vi "rqcBob Initiate.vi"(0 "rqcBob in":refnum<class "rqcBob.lvclass">, 11 "error in (no error)":errorcluster) -> (4 "rqcBob out":refnum<class "rqcBob.lvclass">, 15 "error out":errorcluster)   [LabVIEW 2018, in "rqcBob.lvclass"]
uses:
  rqcBob.lvclass
  rqcBob.lvclass/rqcBob.ctl
  Custom Controls/rqcBob Main FPGA interface.ctl
  Custom Controls/rqcBob State.ctl
  <vilib>/Utility/error.llb/Error Cluster From Error Code.vi
  <vilib>/rvi/errors/niLvFpgaAdjustHostInterfaceError.vi
  <vilib>/rvi/interface/nirviReadWriteControl/nirviReadWriteControl.xnode
  NiFpgaLv.dll
  <vilib>/rvi/interface/Simulation/niFpgaSimulationCallBeginRW.vi
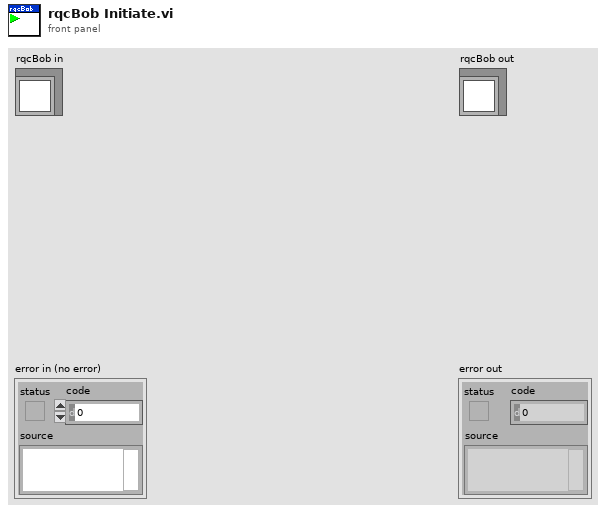
[diagram p1: front panel]
types:
  T1 = typedef "rqcBob.lvclass/rqcBob State.ctl" = enum16{"Idle", "Run"}
  T2 = typedef "rqcBob.lvclass/rqcBob Main FPGA interface.ctl" = refnum<k20>
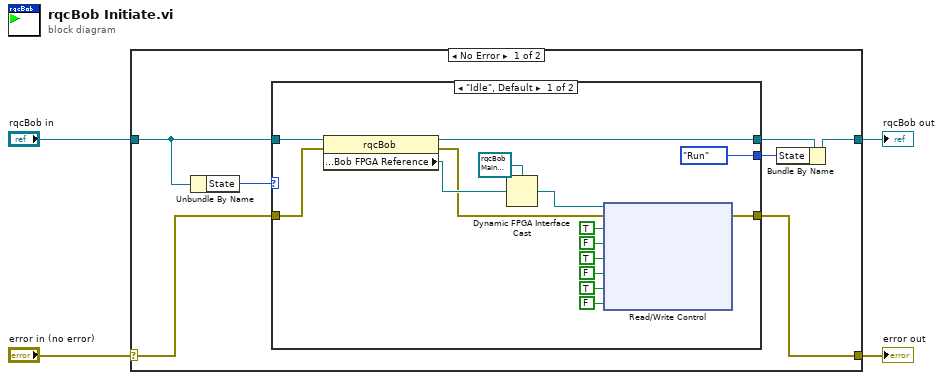
[diagram p0: block diagram]
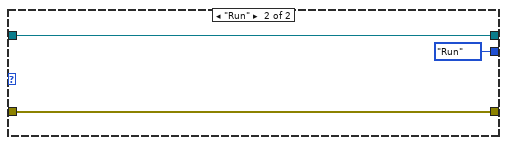
[diagram p2: hidden frame]
diagram:
  n1 = case shown="No Error" "error in (no error)" {
    selector: "error in (no error)" -> [w8 w31]
    tunnel: [w6 w31] -> w3
    tunnel: [w7 w30] -> w1
    tunnel: "rqcBob in" -> [w10 w30]
    frame No Error {
      n2 = Unbundle By Name(w10) -> ("State"=w11:T1)
      n3 = case shown="\"Idle\", Default" w11 {
        tunnel: w10 -> [w26 w29]
        tunnel: [w14 w29] -> w9
        tunnel: w8 -> [w25 w28]
        tunnel: [w13 w28] -> w6
        tunnel: [rqcBob_State."Run" ("State") rqcBob_State."Run" ("State")] -> w5
        frame "Idle", Default {
          n4 = property class="rqcBob"(reference=w26, error in=w25) -> (reference out=w14:refnum<class "rqcBob.lvclass">, error out=w21:errorcluster, "public:Public Properties Access:Bob FPGA Reference"=w23:refnum<k20>)
          n5 = Dynamic FPGA Interface Cast(Session In=T2 refnum ("Bob main FPGA interface"), Type=w23) -> (Session Out=w22:T2)
          n6 = xnode "Read/Write Control"("FPGA VI Reference In"=w22, "error in"=w21, "main.reset"=TRUE, "main.reset"=FALSE, "main.initiate"=TRUE, "main.initiate"=FALSE, "train.software trigger"=TRUE, "train.software trigger"=FALSE) -> ("error out"=w13:errorcluster)  [unwired: 1 out]
        }
        frame "Run" {
        }
      }
      n7 = Bundle By Name(cluster=w9, "State"=w5) -> (w7:refnum<class "rqcBob.lvclass">)
    }
    frame Error {
    }
  }
  "error out" <- w3
  "rqcBob out" <- w1
